vi "read_BJr.vi"   [LabVIEW 2013]
uses:
  <vilib>/NXT/Block Support/NXT_MessageMailbox.ctl
  <vilib>/NXT/Dual Mode Library/Display/drawNumber.vi
  <vilib>/NXT/Dual Mode Library/BT/BlueTooth_Write_Num.vi
  <vilib>/NXT/Dual Mode Library/Sound/Tone.vi
types:
  T1 = typedef "NXT_MessageMailbox.ctl" = u8
  T2 = typedef "LVHSConnector.ctl" = refnum<class "BrickReference.lvclass">
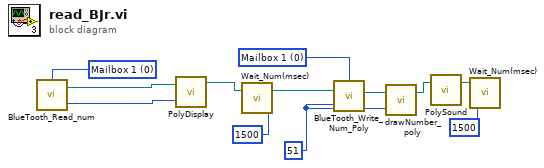
[diagram p0: block diagram]
diagram:
  w8 = T1 0 items=["Mailbox 1", "Mailbox 2", "Mailbox 3", "Mailbox 4", "Mailbox 5", "Mailbox 6", "Mailbox 7", "Mailbox 8", "Mailbox 9", "Mailbox 10"] ("Mailbox")
  w7 = 51 ("Message in")
  w12 = T1 0 items=["Mailbox 1", "Mailbox 2", "Mailbox 3", "Mailbox 4", "Mailbox 5", "Mailbox 6", "Mailbox 7", "Mailbox 8", "Mailbox 9", "Mailbox 10"] ("Mailbox")
  n1 = call <vilib>:"BlueTooth_Read_num.vi"("Mailbox"=w12) -> ("Message"=w11:i32, "NXT/EV3"=w10:T2)  [unwired: 2 in]
  n2 = call-poly <vilib>:"PolyDisplay.vi"("number"=w11, "NXT/EV3"=w10) -> ("NXT/EV3"=w6:T2)  [unwired: 2 in]
  n3 = call <vilib>:"Wait_Num(msec).vi"("Time (100 msec)"=u32 1500, "NXT/EV3"=w6) -> ("NXT/EV3"=w5:T2)  [unwired: 2 in]
  n4 = call-poly <vilib>:"BlueTooth_Write_Num_Poly.vi"("Message"=w7, "NXT/EV3"=w5, "Mailbox"=w8) -> ("NXT/EV3"=w9:T2)  [unwired: 1 in]
  n5 = call-poly <vilib>:"drawNumber_poly.vi"("number"=w7, "NXT/EV3"=w9) -> ("NXT/EV3"=w2:T2)  [unwired: 2 in]
  n6 = call-poly <vilib>:"PolySound.vi"("NXT/EV3"=w2) -> ("NXT/EV3"=w1:T2)  [unwired: 3 in]
  n7 = call <vilib>:"Wait_Num(msec).vi"("Time (100 msec)"=u32 1500, "NXT/EV3"=w1) -> ()  [unwired: 2 in, 1 out]
